vi "Get Elevator Angle.vi"() -> (0 "Elevator Angle":dbl, 1 "Pot Voltage":dbl)   [LabVIEW 2013]
uses:
  Robot Global Data.vi
  <vilib>/addons/control/pid/pid.llb/PID Control Input Filter (DBL).vi
  <vilib>/addons/control/pid/NI_PID_pid.lvlib
panel:
  in  "Pot B":dbl=-65.397
  in  "Pot M":dbl=42.09
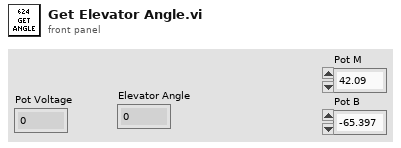
[diagram p1: front panel]
types:
  T1 = typedef "WPI_AnalogChannelDevRef.ctl" = cluster{"DevStatus":errorcluster, "Analog Module":T2, "Analog Channel":T3}
  T2 = typedef "FPGA_TypedefAnalogModule.ctl" = enum16{"Analog Module 1", "Analog Module 2"}
  T3 = typedef "FPGA_AIChannel.ctl" = enum8{"AI 1", "AI 2", "AI 3", "AI 4", "AI 5", "AI 6", "AI 7", "AI 8", "Invalid"}
  T4 = typedef "UDP Dashboard Packet.ctl" = cluster{"Feed Angle":dbl, "Neutral Angle":dbl, "Autonomous Setpoints":T5, "Auto Shift":T6, "Elevator Angle Offset":dbl, "Potentiometer Angle":cluster{"Pot M":dbl, "Pot B":dbl}, "Shoot Setpoints":cluster{"Vision":T7, "Back Corner":T7, "Front":T7, "Front Corner":T7, "Half Court":T7, "Full Court":T7, "Pyramid":T7}, "Halo Drive":T8, "Auto Speed Constants":T9, "Shooting Delays":cluster{"Unjam On":dbl, "Unjam Off":dbl, "Flipper On":dbl, "Flipper Off":dbl, "Hopper Up":dbl}, "Left Roller Pwr":dbl, "Right Roller Pwr":dbl, "Elevator PID Gains":cluster{"proportional gain (Kc)":dbl, "integral time (Ti, min)":dbl, "derivative time (Td, min)":dbl}, "Elevator PID Output Range":cluster{"output high":dbl, "output low":dbl}, "Elevator Angle Tolerance":dbl, "Toggle Ears Delay":dbl, "Toggle Ears Distance":dbl, "Unjam Servo Angle":dbl, "Auton Steer PID gains":cluster{"proportional gain (Kc)":dbl, "integral time (Ti, min)":dbl, "derivative time (Td, min)":dbl}, "Auton Steer output range":cluster{"output high":dbl, "output low":dbl}, "Auto Reverse Speed":dbl, "Auto Stop Throttle":dbl, "Auto Stop Duration":dbl, "Spin output range":cluster{"output high":dbl, "output low":dbl}, "Spin PID gains":cluster{"proportional gain (Kc)":dbl, "integral time (Ti, min)":dbl, "derivative time (Td, min)":dbl}, "Auto-Center Line":T10, "Auton Distance PID gains Low Gear":cluster{"proportional gain (Kc)":dbl, "integral time (Ti, min)":dbl, "derivative time (Td, min)":dbl}, "Auton Distance output range":cluster{"output high":dbl, "output low":dbl}, "Auton Distance Threshold":dbl, "Auton Velocity Cutoff":dbl, "Auton Distance output range Center Line":cluster{"output high":dbl, "output low":dbl}, "Auton Distance PID gains High Gear":cluster{"proportional gain (Kc)":dbl, "integral time (Ti, min)":dbl, "derivative time (Td, min)":dbl}}
  T5 = typedef "Autonomous Setpoints.ctl" = cluster{"Shoot Angle 1":dbl, "Initial Delay":dbl, "Disc Count 1":dbl, "Shoot Time 1":dbl, "Distance 1":dbl, "Two Disc Distance 1":dbl, "Distance 2":dbl, "Two Disc Distance 2":dbl, "Distance 3":dbl, "Two Disc Distance 3":dbl, "Shoot Angle 3":dbl, "Disc Count 3":dbl, "Shoot Time 3":dbl, "Distance 4":dbl, "Two Disc Distance 4":dbl, "Low Gear":bool, "Shoot 1 Post Delay":dbl}
  T6 = typedef "Auto Shift Settings.ctl" = cluster{"Enabled":bool, "Upshift Speed":dbl, "Downshift Speed":dbl, "Upshift Throttle":dbl, "Turn Power Diff":dbl, "Motor Limit":dbl, "Encoder Limit":dbl}
  T7 = typedef "Shoot Profile.ctl" = cluster{"Pre RPM":dbl, "Main RPM":dbl, "Angle":dbl}
  T8 = typedef "Halo Drive.ctl" = cluster{"Gains":cluster{"Quickturn_Sens_Low":dbl, "Quickturn_Sens_High":dbl, "Speedturn_Sens_Low":dbl, "Speedturn_Sens_High":dbl}, "QuickTurn Const":dbl, "Loading Throttle Limit":dbl}
  T9 = typedef "Auto Speed Constants.ctl" = cluster{"Slowing Distance":dbl, "High Speed":dbl, "Rampup Time":dbl, "Low Speed":dbl, "High Speed (Reverse)":dbl}
  T10 = typedef "Autonomous Center Line Setpoints.ctl" = cluster{"Arc Turn x-axis":dbl, "Arc Turn y-axis":dbl, "Arc Turn Distance":dbl, "Distance 1":dbl, "Two Disc Distance 1":dbl, "Distance 2":dbl, "Two Disc Distance 2":dbl, "Spin Angle":dbl, "Spin Angle tolerance":dbl, "Spin y-axis":dbl, "Spin Distance":dbl, "Center Line Enabled":bool, "Distance 3":dbl, "Two Disc Distance 3":dbl, "Spin Angle 2":dbl, "Spin Angle tolerance 2":dbl, "Spin y-axis 2":dbl, "Spin Distance 2":dbl, "Shoot Angle 1":dbl, "Disc Count 1":dbl, "Shoot Time 1":dbl, "Shoot Angle 3":dbl, "Disc Count 3":dbl, "Shoot Time 3":dbl, "Low Gear":bool}
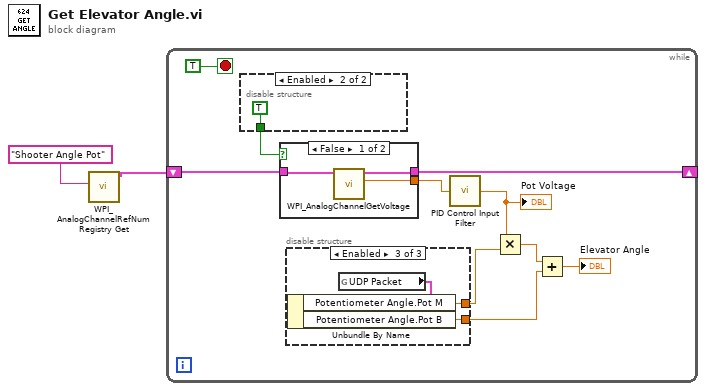
[diagram p0: block diagram]
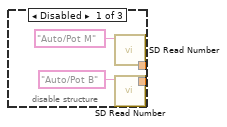
[diagram p2: hidden frame]
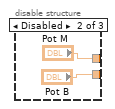
[diagram p3: hidden frame]
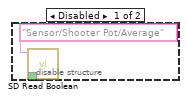
[diagram p4: hidden frame]
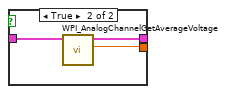
[diagram p5: hidden frame]
diagram:
  n1 = call <vilib>:"WPI_AnalogChannelRefNum Registry Get.vi"("refnum name"="Shooter Angle Pot") -> ("AIDeviceRef"=w1:T1)  [unwired: 9 in, 1 out]
  n2 = while {
    shift-right: [w11] -> _
    shift-left: w1 -> [w6]
    stop <- TRUE stop-if-true
    n3 = disable-structure shown="Enabled" {
      disable-tunnel: [w22 TRUE ("Boolean")] -> w12
      frame Disabled {
        n4 = call <vilib>:"SD Read Boolean.vi"("Name"="Sensor/Shooter Pot/Average") -> ("Boolean"=w22:bool)  [unwired: 8 in, 2 out]
      }
      frame Enabled {
      }
    }
    n5 = case shown="False" w12 {
      tunnel: [w27 w30] -> w11
      tunnel: [w26 w29] -> w3
      tunnel: w6 -> [w25 w28]
      frame False {
        n6 = call <vilib>:"WPI_AnalogChannelGetVoltage.vi"("AIDeviceRef"=w25) -> ("Voltage"=w26:dbl, "AIDeviceRef"=w27:T1)  [unwired: 8 in, 1 out]
      }
      frame True {
        n7 = call <vilib>:"WPI_AnalogChannelGetAverageVoltage.vi"("AIDeviceRef"=w28) -> ("Voltage"=w29:dbl, "AIDeviceRef"=w30:T1)  [unwired: 8 in, 1 out]
      }
    }
    n8 = disable-structure shown="Enabled" {
      disable-tunnel: [w16 "Pot B" w19] -> w9
      disable-tunnel: [w15 "Pot M" w20] -> w8
      frame Disabled {
        n9 = call <vilib>:"SD Read Number.vi"("Name"="Auto/Pot M") -> ("Numeric"=w15:dbl)  [unwired: 8 in, 2 out]
        n10 = call <vilib>:"SD Read Number.vi"("Name"="Auto/Pot B") -> ("Numeric"=w16:dbl)  [unwired: 8 in, 2 out]
      }
      frame Disabled {
      }
      frame Enabled {
        n11 = global read "Robot Global Data.vi" "UDP Packet"() -> (w21:T4)
        n12 = Unbundle By Name(w21) -> ("Potentiometer Angle.Pot M"=w20:dbl, "Potentiometer Angle.Pot B"=w19:dbl)
      }
    }
    n13 = call-poly <vilib>:"PID Control Input Filter.vi"("input"=w3) -> ("output"=w4:dbl)  [unwired: 4 in]
    "Pot Voltage" <- w4
    n14 = Multiply(x=w4, y=w8) -> (x*y=w7:dbl)
    n15 = Add(x=w7, y=w9) -> (x+y=→"Elevator Angle":dbl)
  }
